vi "Chirp_EIS_Measurement.vi"(8 "error in (no error)":errorcluster, 11 "ChirpEIS in":refnum<class "ChirpEIS.lvclass">) -> (0 "error out":errorcluster, 1 "Experiment Variables.DC_Bias":dbl, 2 "data":dynamicdata(graph), 3 "ChirpEIS out":refnum<class "ChirpEIS.lvclass">, 4 "data 2":waveform(dbl)(graph) caption="Superinposed Chirp")   [LabVIEW 2014, in "ChirpEIS.lvclass"]
uses:
  ChirpEIS.lvclass
  ChirpEIS.lvclass/ChirpEIS.ctl
  <vilib>/addons/_NISVFA/_Generation/SoundVib_Generation.lvlib
  <vilib>/measure/NI_MABase.lvlib
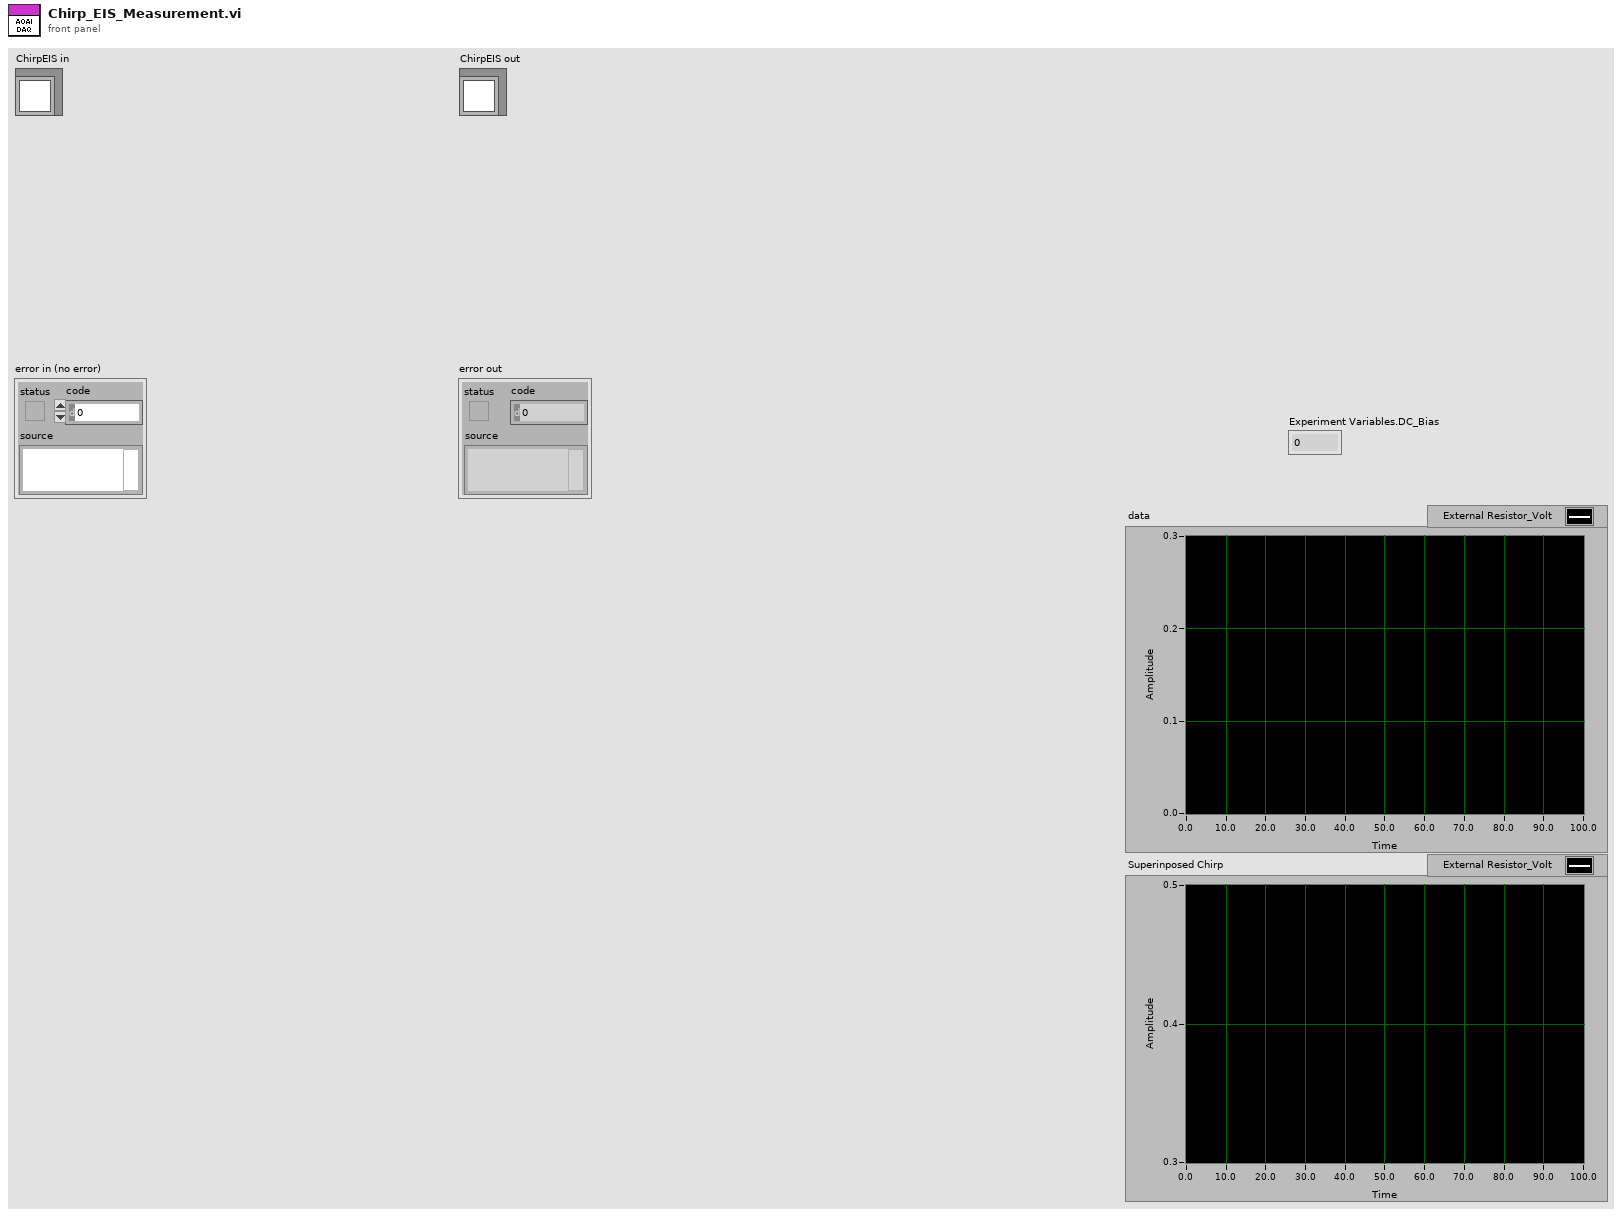
[diagram p1: front panel]
types:
  T1 = cluster{"start frequency [Hz]":dbl, "stop frequency [Hz]":dbl}
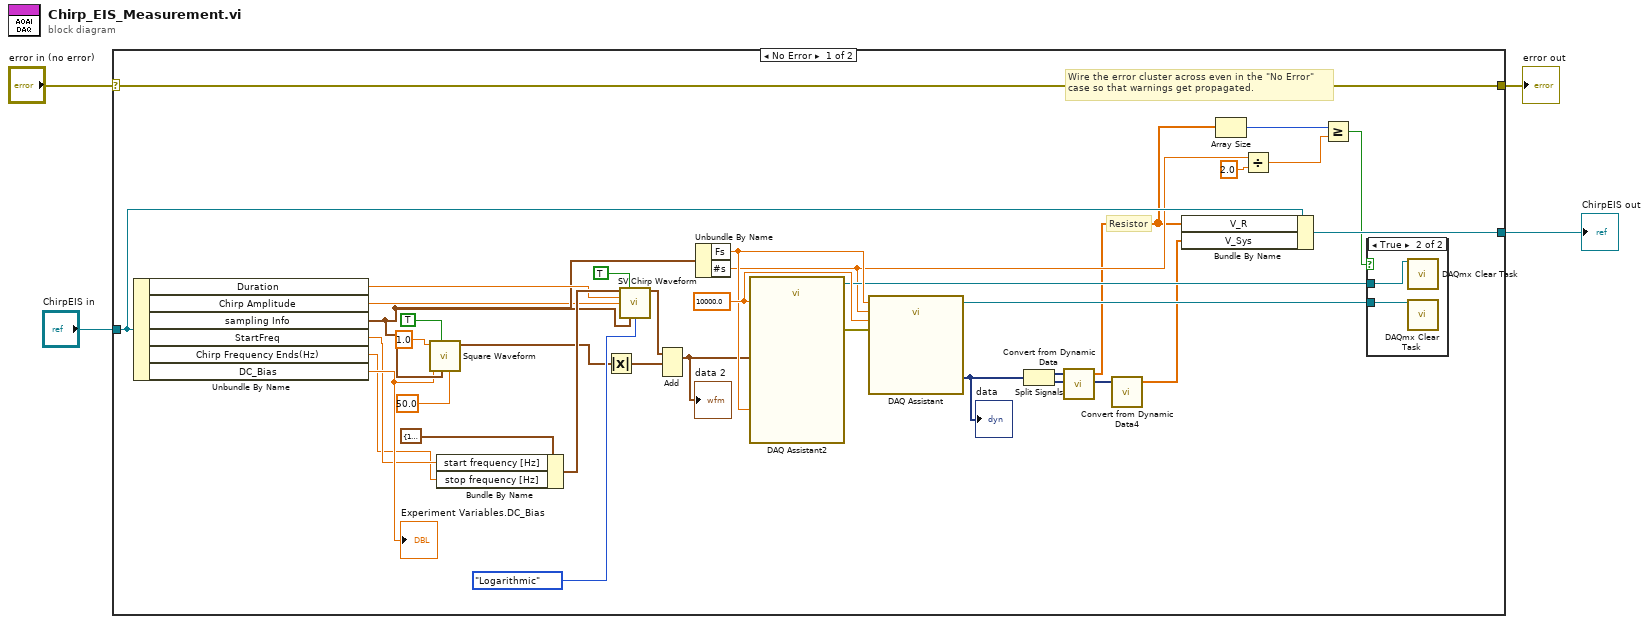
[diagram p0: block diagram]
diagram:
  n1 = case shown="No Error" "error in (no error)" {
    selector: "error in (no error)" -> [w39 w43]
    tunnel: [w39 w43] -> w3
    tunnel: [w22 w42] -> w1
    tunnel: "ChirpEIS in" -> [w21 w42]
    frame No Error {
      w35 = 10000.0 ("timeout (s)")
      # "Resistor"
      # "Wire the error cluster across even in the \"No Error\"\ncase so that warnings get propagated."
      n2 = Unbundle By Name(w21) -> ("Duration"=w25:dbl, "Chirp Amplitude"=w14:dbl, "sampling Info"=w24:cluster{"Fs":dbl, "#s":dbl}, "StartFreq"=w6:dbl, "Chirp Frequency Ends(Hz)"=w5:dbl, "DC_Bias"=w12:dbl)
      "Experiment Variables.DC_Bias" <- w12
      n3 = call <vilib>:"Square Waveform.vi"("duty cycle (%)"=50.0, "sampling info"=w24, "reset signal"=TRUE, "amplitude"=w12, "frequency"=1.0) -> ("signal out"=w29:waveform(dbl))  [unwired: 5 in, 1 out]
      n4 = Bundle By Name(cluster=T1 {"start frequency [Hz]"=10.0, "stop frequency [Hz]"=10000.0} ("frequency range"), "start frequency [Hz]"=w6, "stop frequency [Hz]"=w5) -> (w36:T1)
      n5 = Absolute Value(x=w29) -> (abs(x)=w10:waveform(dbl))
      n6 = call <vilib>:"SV Chirp Waveform.vi"("frequency range"=w36, "reset signal (F)"=TRUE, "chirp duration [s]"=w25, "amplitude"=w14, "sampling info"=w24, "frequency spacing"=enum16{"Linear", "Logarithmic"}."Logarithmic") -> ("chirp signal"=w8:waveform(dbl))  [unwired: 7 in, 2 out]
      n7 = Add(1:w10, 2:w8) -> (0:w9:waveform(dbl))  [unwired: 1 in, 1 out]
      "data 2" <- w9
      n8 = Unbundle By Name(w24) -> ("Fs"=w34:dbl, "#s"=w18:dbl)
      n9 = call "DAQ Assistant2"("data"=w9, "rate"=w34, "timeout (s)"=w35) -> ("task out"=w31:refnum<k21>, "error out"=w11:errorcluster)  [unwired: 14 in, 1 out]
      n10 = call "DAQ Assistant"("rate"=w34, "number of samples"=w18, "timeout (s)"=w35, "error in"=w11) -> ("task out"=w32:refnum<k21>, "data"=w28:dynamicdata)  [unwired: 13 in, 1 out]
      "data" <- w28
      n11 = Split Signals(w28) -> (w27:dynamicdata, w7:dynamicdata)  [unwired: 2 in]
      n12 = call "Convert from Dynamic Data"("Dynamic Data Type"=w27) -> ("Array"=w15:dbl[])  [unwired: 3 in]
      n13 = call "Convert from Dynamic Data4"("Dynamic Data Type"=w7) -> ("Array"=w23:dbl[])  [unwired: 3 in]
      n14 = Bundle By Name(cluster=w21, "V_R"=w15, "V_Sys"=w23) -> (w22:refnum<class "ChirpEIS.lvclass">)
      n15 = Array Size(array=w15) -> (size(s)=w20:i32)
      n16 = Divide(x=w18, y=2.0) -> (x/y=w16:dbl)
      n17 = Greater Or Equal?(x=w20, y=w16) -> (x >= y?=w19:bool)
      n18 = case shown="True" w19 {
        tunnel: w32 -> [_ w41]
        tunnel: w31 -> [_ w40]
        frame False {
        }
        frame True {
          n19 = call <vilib>:"DAQmx Clear Task.vi"("task in"=w40) -> ()  [unwired: 14 in, 1 out]
          n20 = call <vilib>:"DAQmx Clear Task.vi"("task in"=w41) -> ()  [unwired: 14 in, 1 out]
        }
      }
    }
    frame Error {
    }
  }
  "error out" <- w3
  "ChirpEIS out" <- w1
